vi "NF WF1973_74 MEM Del.vi"(8 "error in (no error)":errorcluster caption="Error IN", 10 "Memory No(1)":i32(knob)=1 min=1 max=10 step=1 scale=1.0..10.0, 11 "VISAsession":refnum<visa-resource-name>) -> (0 "error out":errorcluster caption="Error OUT", 3 "CopyVISAsession":refnum<visa-resource-name>)   [LabVIEW 2010]
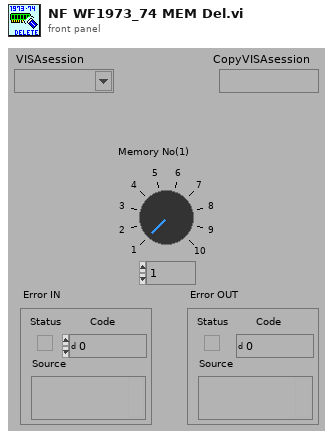
[diagram p1: front panel]
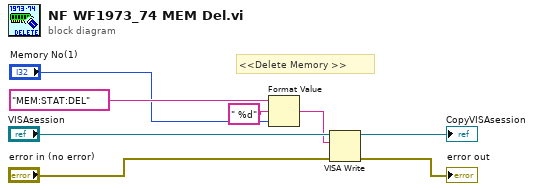
[diagram p0: block diagram]
diagram:
  # "<<Delete Memory >>"
  n1 = Format Value(string ("")="MEM:STAT:DEL" ("文字列"), format string=" %d" ("形式文字列"), value (0)="Memory No(1)") -> (output string=w1:string)
  n2 = VISA Write(VISA resource name="VISAsession", write buffer=w1, error in (no error)="error in (no error)") -> (VISA resource name out=→"CopyVISAsession":refnum<visa-resource-name>, error out=→"error out":errorcluster)  [unwired: 1 out]
